vi "XML Get First Child Value.vi"(0 "XML Ref In":refnum<k20>, 5 "Tag Name":string, 11 "error in (no error)":errorcluster) -> (4 "XML Ref Out":refnum<k20>, 6 "Node Value":string, 15 "error out":errorcluster)   [LabVIEW 2017, in "CL_G3_VIPMUtilities.lvlib"]
doc: "Gets the first child node value of the specified tag"
uses:
  CL_G3_VIPMUtilities.lvlib
  <vilib>/xml/Close Reference(Node).vi
  <vilib>/xml/Close Reference(NdList).vi
  <resource>/objmgr/DOMUserDefRef.rc
  <vilib>/xml/NI_XML.lvlib
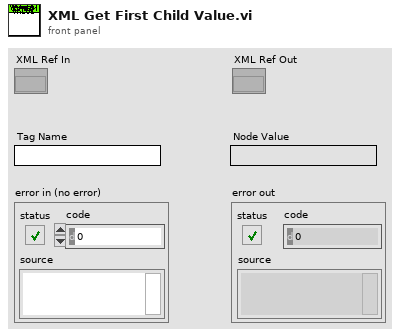
[diagram p1: front panel]
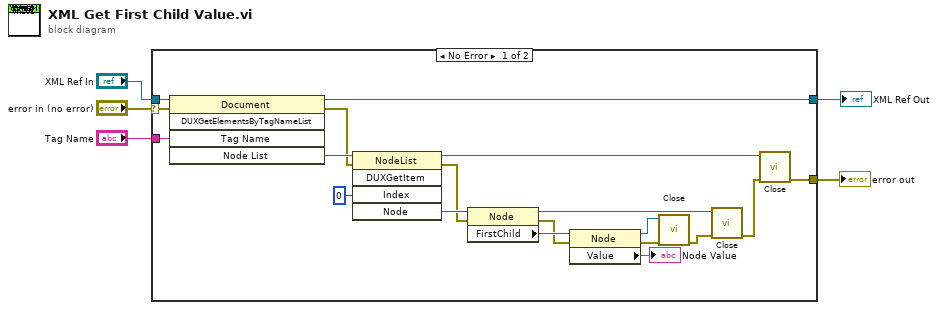
[diagram p0: block diagram]
diagram:
  n1 = case shown="No Error" "error in (no error)" {
    selector: "error in (no error)" -> [w9 w26]
    tunnel: "Tag Name" -> [w10 _]
    tunnel: "XML Ref In" -> [w8 w25]
    tunnel: [w7 w25] -> w2
    tunnel: [w6 w26] -> w1
    frame No Error {
      n2 = invoke class="Document" method="DUXGetElementsByTagNameList"(reference=w8, error in=w9, "Tag Name"=w10) -> (reference out=w7:refnum<k20>, error out=w20:errorcluster, "Node List"=w24:refnum<k20>)  [unwired: 2 in, 2 out]
      n3 = invoke class="NodeList" method="DUXGetItem"(reference=w24, error in=w20, "Index"=0) -> (reference out=w13:refnum<k20>, error out=w19:errorcluster, "Node"=w22:refnum<k20>)  [unwired: 2 in, 2 out]
      n4 = property class="Node"(reference=w22, error in=w19) -> (reference out=w14:refnum<k20>, error out=w18:errorcluster, "FirstChild"=w21:refnum<k20>)
      n5 = property class="Node"(reference=w21, error in=w18) -> (reference out=w16:refnum<k20>, error out=w17:errorcluster, "Value"=→"Node Value":string)
      n6 = call-poly <vilib>:"Close.vi"("error in (no error)"=w17, "node"=w16) -> ("error out"=w15:errorcluster)  [unwired: 7 in]
      n7 = call-poly <vilib>:"Close.vi"("error in (no error)"=w15, "node"=w14) -> ("error out"=w12:errorcluster)  [unwired: 7 in]
      n8 = call-poly <vilib>:"Close.vi"("error in (no error)"=w12, "node list"=w13) -> ("error out"=w6:errorcluster)  [unwired: 7 in]
    }
    frame Error {
    }
  }
  "error out" <- w1
  "XML Ref Out" <- w2
